vi "Get_Keys.vi"(0 "Target_Data":map{string, refnum<class "I2C.lvclass">}(c390)) -> (4 "Keys_and_Index":cluster{"String":string, "Value":u16}[](array[cluster]), 6 "Keys":string[](array[string]))   [LabVIEW 2023]
uses:
  Class/I2C/I2C.lvclass
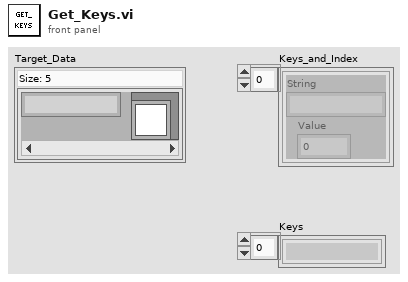
[diagram p1: front panel]
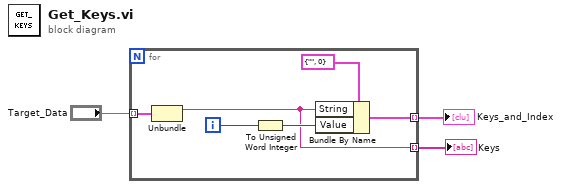
[diagram p0: block diagram]
diagram:
  n1 = for {
    tunnel: [w7] -> w3 mode=indexing
    tunnel: "Target_Data" -> [w6] mode=indexing
    tunnel: [w4] -> w1 mode=indexing
    i -> [w8]
    n2 = Unbundle(w6) -> (w4:string)  [unwired: 1 out]
    n3 = To Unsigned Word Integer(number=w8) -> (unsigned 16bit integer=w5:u16)
    n4 = Bundle By Name(cluster=cluster{"String":string, "Value":u16} {"String"="", "Value"=0} ("Cluster"), "String"=w4, "Value"=w5) -> (w7:cluster{"String":string, "Value":u16})
  }
  "Keys_and_Index" <- w3
  "Keys" <- w1
